vi "Clip-Ball_Test.vi"() -> ()   [LabVIEW 2019]
uses:
  <vilib>/myRIO/Instrument Drivers/Utilities/Utilities.lvlib
panel:
  out "Error Out":errorcluster
  in  "Error In":errorcluster
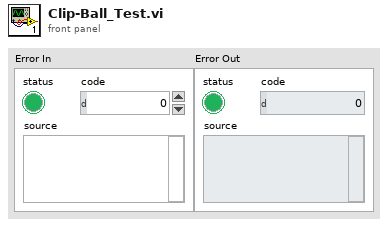
[diagram p1: front panel]
types:
  T1 = typedef "I2C.lvlib/I2C Reference.ctl" = cluster{"myRIO Reference":T2, "I2C Channels Enum":T6, "I2C Configuration":T7}
  T2 = typedef "myRIO Generic Hardware Reference.ctl" = cluster{"myRIO Model":T3, "myRIO Hardware Reference":T4}
  T3 = typedef "Hardware Version Enum.ctl" = enum16{"Unknown", "myRIO-1900", "myRIO-1950", "roboRIO", "NI ELVIS RIO CM", "ELVIS III"}
  T4 = typedef "myRIO v1.0 Reference.ctl" = cluster{"Generic FPGA Reference":T5, "Allow multiple opens":bool}
  T5 = typedef "Generic FPGA Reference.ctl" = refnum<k20>
  T6 = typedef "I2C Channels Enum.ctl" = enum16{"Not Connected", "A/I2C", "B/I2C", "I2C/I2C"}
  T7 = typedef "I2C.lvlib/I2C Configuration.ctl" = cluster{"I2C Transfer Rate":T8}
  T8 = typedef "I2C.lvlib/I2C Transfer Rate.ctl" = enum16{"Standard mode (100 kbps)", "Fast mode (400 kbps)"}
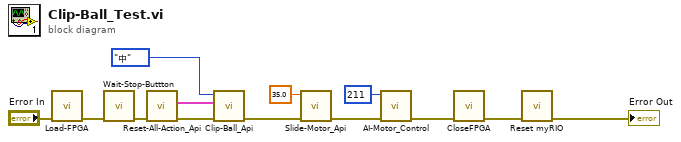
[diagram p0: block diagram]
diagram:
  n1 = call "Load-FPGA.vi"("Error In"="Error In") -> ("Error Out"=w12:errorcluster)  [unwired: 10 in]
  n2 = call "Wait-Stop-Buttton.vi"("Error In"=w12) -> ("Error Out"=w10:errorcluster)  [unwired: 10 in]
  n3 = call "Reset-All-Action_Api.vi"("Error In"=w10) -> ("Error Out"=w9:errorcluster, "I2C Ref Out"=w7:T1)  [unwired: 8 in, 1 out]
  n4 = call "Clip-Ball_Api.vi"("Error In"=w9, 10:w7, "動作"=enum16{"オ", "中", "右"}."中" ("夾爪組合?")) -> ("Error Out"=w6:errorcluster)  [unwired: 8 in]
  n5 = call "Slide-Motor_Api.vi"("Error In"=w6, "移動距離"=35.0) -> ("Error Out"=w4:errorcluster)  [unwired: 9 in]
  n6 = call "AI-Motor_Control.vi"("Error In"=w4, "目標位置(0~4095)"=u16 211) -> ("Error Out"=w2:errorcluster)  [unwired: 9 in]
  n7 = call "CloseFPGA.vi"("Error In"=w2) -> ("Error Out"=w13:errorcluster)  [unwired: 10 in]
  n8 = call <vilib>:"Reset myRIO.vi"("error in (no error)"=w13) -> ("error out"=→"Error Out":errorcluster)  [unwired: 10 in]
